vi "Pico3-1pulse.vi"(5 "+ ou -":bool, 7 "sélecteur":bool, 11 "DataIn":cluster{"Rch":dbl, "A ch":dbl, "max":dbl}) -> (2 "Rout":string, 3 "Chaîne":string)   [LabVIEW 2020]
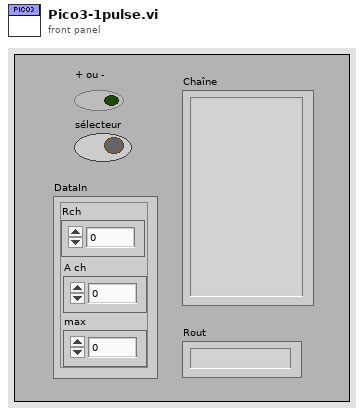
[diagram p1: front panel]
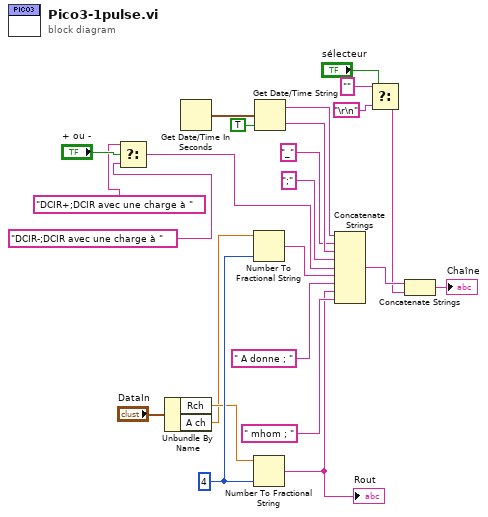
[diagram p0: block diagram]
diagram:
  w24 = i16 4 ("précision (6)")
  n1 = Select(t="DCIR+;DCIR avec une charge à " ("chaîne"), s="+ ou -", f="DCIR-;DCIR avec une charge à " ("chaîne")) -> (s? t:f=w3:string)
  n2 = Unbundle By Name("DataIn") -> ("Rch"=w12:dbl, "A ch"=w11:dbl)
  n3 = Get Date/Time In Seconds() -> (seconds since 1Jan1904=w18:timestamp)
  n4 = Number To Fractional String(number=w11, precision (6)=w24) -> (F-format string=w23:string)  [unwired: 2 in]
  n5 = Number To Fractional String(number=w12, precision (6)=w24) -> (F-format string=w5:string)  [unwired: 2 in]
  "Rout" <- w5
  n6 = Get Date/Time String(seconds (now)=w18, want seconds? (F)=TRUE ("secondes ? (F)")) -> (date string=w14:string, time string=w16:string)  [unwired: 1 in]
  n7 = Concatenate Strings(w14, "_" ("chaîne"), w16, ";" ("chaîne"), w3, w23, " A donne ; " ("chaîne"), w5, " mhom ; " ("chaîne")) -> (w19:string)
  n8 = Select(t="" ("cas vrai"), s="sélecteur", f="\r\n") -> (s? t:f=w8:string)
  n9 = Concatenate Strings(w19, w8) -> (→"Chaîne":string)
